vi "LS370 Change Excitation Com edit.vi"(1 "command text in":string[](array[string])) -> (0 "Command text out":string[][](array[string]))   [LabVIEW 2019]
uses:
  LS370 Excitation Voltage.ctl
  LS370 Resistance Range.ctl
  LS370 Excitation Current.ctl
panel:
  in  "Current":T1
  in  "Mode":enum32{"Voltage", "Current"}(radio)
  in  "VISA Resource Name":refnum<visa-resource-name> caption="VISA Name"
  in  "Resistance Range":T2
  in  "enter":bool
  in  "extra wait":i32 min=0
  in  "Channel":i32=1 min=1 max=16 step=1
  in  "Voltage":T3
  in  "cancel":bool
  # "seconds"
  # "AND wait extra"
  # "LakeShore 370 Change Excitation"
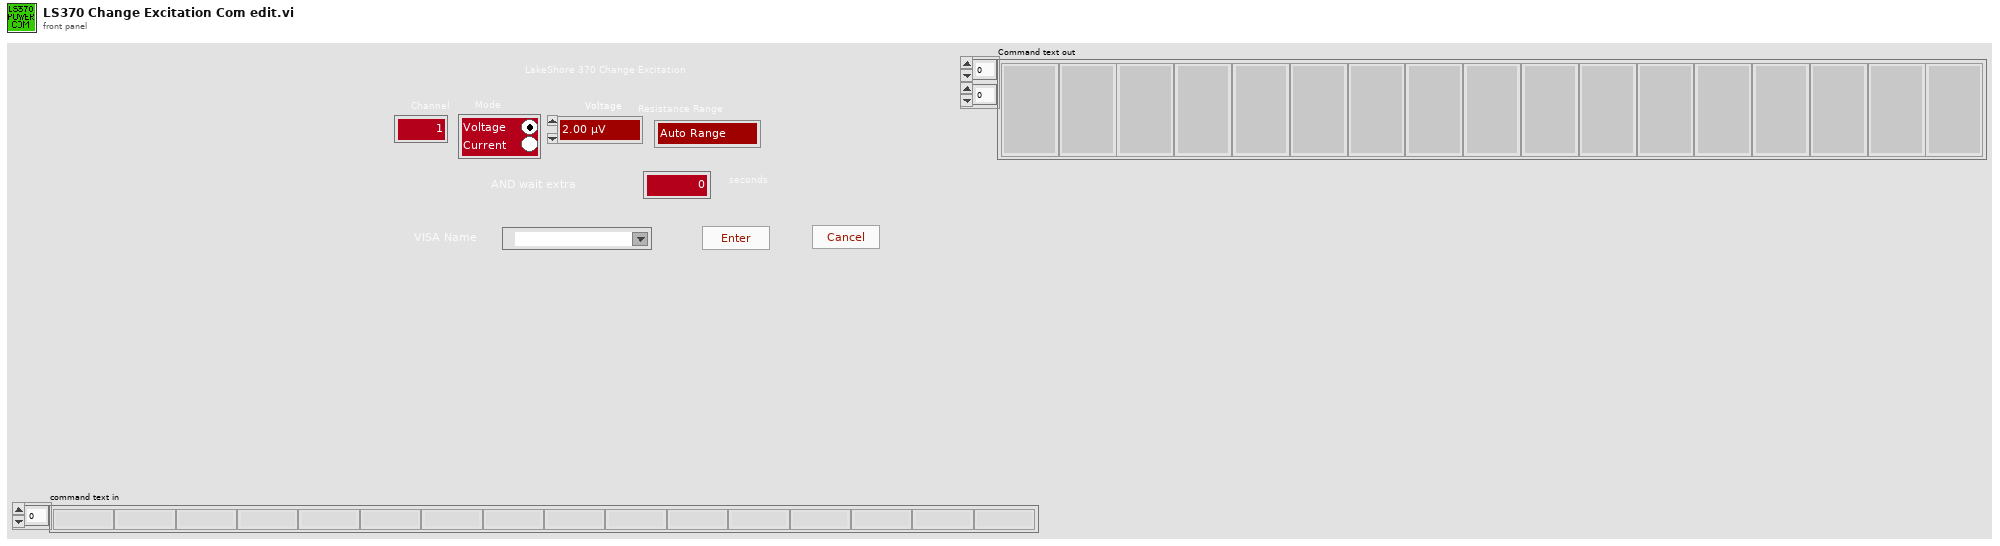
[diagram p1: front panel]
types:
  T1 = typedef "LS370 Excitation Current.ctl" = enum16{"1.00 pA", "3.16 pA", "10.0 pA", "31.6 pA", "100 pA", "316 pA", "1.00 nA", "3.16 nA", "10.0 nA", "31.6 nA", "100 nA", "316 nA", "1.00 µA", "3.16 µA", "10.0 µA", "31.6 µA", "100 µA", "316 µA", "1.00 mA", "3.16mA", "10.0 mA", "31.6 mA"}
  T2 = typedef "LS370 Resistance Range.ctl" = enum16{"Auto Range", "2.00 mΩ", "6.32 mΩ", "20.0 mΩ", "63.2 mΩ", "200 mΩ", "632 mΩ", "2.00 Ω", "6.32 Ω", "20.0 Ω", "63.2 Ω", "200 Ω", "632 Ω", "2.00 kΩ", "6.32 kΩ", "20.0 kΩ", "63.2 kΩ", "200 kΩ", "632 kΩ", "2.00 MΩ", "6.32 MΩ", "20.0 MΩ", "63.2 MΩ"}
  T3 = typedef "LS370 Excitation Voltage.ctl" = enum16{"2.00 µV", "6.32 µV", "20.0 µV", "63.2 µV", "200 µV", "632 µV", "2.00 mV", "6.32 mV", "20.0 mV", "63.2 mV", "200 mV", "632 mV"}
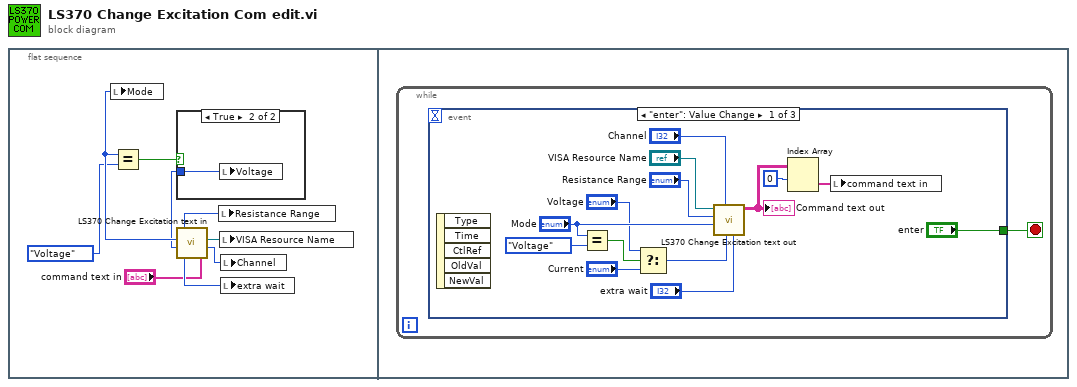
[diagram p0: block diagram]
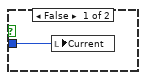
[diagram p2: hidden frame]
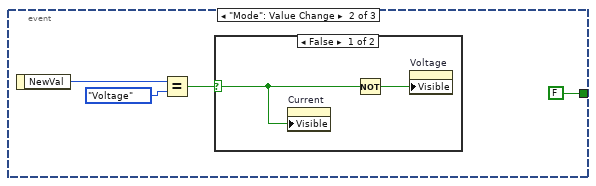
[diagram p3: hidden frame]
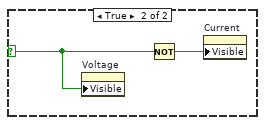
[diagram p4: hidden frame]
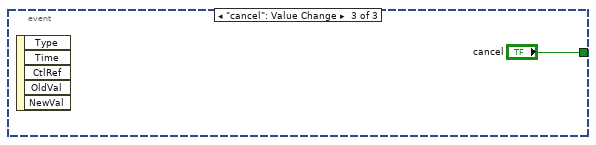
[diagram p5: hidden frame]
diagram:
  n1 = flat-sequence {
    frame #0 {
      n2 = call "LS370 Change Excitation text in.vi"("command text in"="command text in") -> ("Channel"=w7:i32, "VISA Refnum in"=w9:refnum<visa-resource-name>, "extra wait"=w8:i32, "Current"=w2:u16, "Mode"=w6:enum32{"Voltage", "Current"}, "Resistance Range"=w4:T2)  [unwired: 1 out]
      n3 = local write "Mode"(w6) -> ()
      n4 = Equal?(x=w6, y=enum32{"Voltage", "Current"}."Voltage") -> (x = y?=w3:bool)
      n5 = case shown="True" w3 {
        tunnel: w2 -> [w10 w11]
        frame False {
          n6 = local write "Current"(w10) -> ()
        }
        frame True {
          n7 = local write "Voltage"(w11) -> ()
        }
      }
      n8 = local write "Resistance Range"(w4) -> ()
      n9 = local write "VISA Resource Name"(w9) -> ()
      n10 = local write "Channel"(w7) -> ()
      n11 = local write "extra wait"(w8) -> ()
    }
    frame #1 {
      n12 = while {
        stop <- w12 stop-if-true
        n13 = event shown="[0] \"enter\": Value Change" {
          selector: _ -> [_ _ _]
          dyn-events: _ -> [_ _ _]
          timeout: _ -> [_ _ _]
          tunnel: ["enter" FALSE ("cancel") "cancel"] -> w12
          event "enter": Value Change {
            n14 = event-data() -> ()  [unwired: 1 in, 5 out]
            n15 = Equal?(x="Mode", y=enum32{"Voltage", "Current"}."Voltage") -> (x = y?=w19:bool)
            n16 = Select(t="Voltage", s=w19, f="Current") -> (s? t:f=w18:u16)
            n17 = call "LS370 Change Excitation text out.vi"("extra wait"="extra wait", "Current"=w18, "Channel"="Channel", "Mode"="Mode", "Resistance Range"="Resistance Range", "VISA Refnum in"="VISA Resource Name") -> ("Command text"=w15:string[][])  [unwired: 5 in]
            "Command text out" <- w15
            n18 = Index Array(array=w15, index (row)=0) -> (element=w16:string[])  [unwired: 1 in]
            n19 = local write "command text in"(w16) -> ()
          }
          event "Mode": Value Change {
            n20 = event-data() -> ("NewVal"=w30:enum32{"Voltage", "Current"})  [unwired: 1 in]
            n21 = Equal?(x=w30, y=enum32{"Voltage", "Current"}."Voltage") -> (x = y?=w28:bool)
            n22 = case shown="False" w28 {
              selector: w28 -> [w31 w34]
              frame False {
                n23 = property on="Current" class="Enum (strict)"("Visible"=w31) -> ()  [unwired: 2 in, 2 out]
                n24 = Not(x=w31) -> (.not. x?=w32:bool)
                n25 = property on="Voltage" class="Enum (strict)"("Visible"=w32) -> ()  [unwired: 2 in, 2 out]
              }
              frame True {
                n26 = property on="Voltage" class="Enum (strict)"("Visible"=w34) -> ()  [unwired: 2 in, 2 out]
                n27 = Not(x=w34) -> (.not. x?=w33:bool)
                n28 = property on="Current" class="Enum (strict)"("Visible"=w33) -> ()  [unwired: 2 in, 2 out]
              }
            }
          }
          event "cancel": Value Change {
            n29 = event-data() -> ()  [unwired: 1 in, 5 out]
          }
        }
      }
    }
  }
